vi "niFpgaWaitForSimulatedTimeMergeVi.vi"   [LabVIEW 2017]
doc: "Waits for the time you specify. For example, you can use this VI to debug a problem that occurs at a specific time in the simulation or to allow simulation time to advance while the LabVIEW test bench runs."
uses:
  <vilib>/FPGA/simulation/niFpgaWaitForSimulatedTimeNs.vi
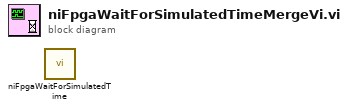
[diagram p0: block diagram]
diagram:
  n1 = call-poly <vilib>:"niFpgaWaitForSimulatedTime.vi"() -> ()  [unwired: 10 in, 2 out]
